vi "PH_BeamlineController.constructor.vi"(0 "name":string, 2 "data in":string, 5 "error in(no error)":errorcluster) -> (14 "i ref out":refnum<vi>, 16 "data out":string, 19 "error out":errorcluster)   [LabVIEW 2014, in "PH_BeamlineController.lvlib"]
doc: "The Sequencer controlles the PHELIX shot procedure.\n\nThis class is part of the PHELIX user layer.\n\nauthor: Stefan Götte, GSI\n\nLicense Agreement for this software:\n\nCopyright (C)\nGesellschaft für Schwerionenforschung, GSI\nPlanckstr. 1\n64291 Darmstadt\nGermany\n\nContact: D.Beck@gsi.de \n\nThis program is free software; you can redistribute it and/or modify it under the terms of the \nGNU General Public License as published by the Free Software Foundation; either version 2 of \nthe license, or (at your option) any later version.\n\nThis program is distributed in the hope that it will be useful, but WITHOUT ANY WARRANTY; \nwithout even the implied warranty of MERCHANTABILITY or FITNESS FOR A PARTICULAR PURPOSE. See the GNU General License for more details (http://www.gnu.org).\n\nGesellschaft für Schwerionenforschung, GSI\nPlanckstr. 1, 64291 Darmstadt, Germany\nFor all questions and ideas contact: M.Richter@gsi.de, H.Brand@gsi.de or D.Beck@gsi.de.\nLast update: 16-JUN-2004"
uses:
  PH_BeamlineController.lvlib
  PH_BeamlineInformation/PH_BeamlineInformation.lvlib
  CS_Core/CSSystem/CSSystemLib/CSSystemLib.lvlib
  PH_Basics/PH_Class/PH_Class.lvlib
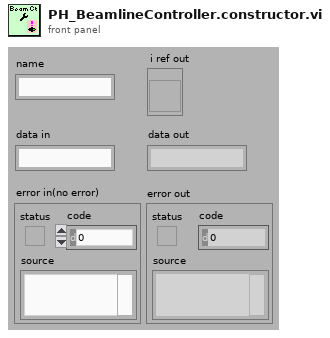
[diagram p1: front panel]
types:
  T1 = enum16{"SetAttribute", "GetAttribute", "CreateAttribute", "DestroyAttribute", "DestroyAllAtributes"}
  T2 = typedef "PH_BeamlineController.lvlib/PH_BeamlineController.i attribute.ctl" = cluster{"Vacuum Exp LB":cluster{"Channel":string, "Limit [mbar]":dbl, "Pressure [mbar]":dbl, "GUI Ref":refnum<vi>}, "Sources":T3[], "PA DP Targets":T5[], "Path":cluster{"Source":T4, "PA DP Target":T6, "Target":T7}, "Targets":cluster{"Name":T7, "GUI Ref":refnum<vi>, "Current State":bool, "Wanted State":bool, "Enabled":bool}[], "Status Tags":cluster{"Name":string, "Status":T8}[], "special GUI Refs":T9}
  T3 = typedef "PH_BeamlineController.lvlib/PH_BeamlineController.Source Attributes.ctl" = cluster{"Name":T4, "GUI Ref":refnum<vi>, "Current State":bool, "Wanted State":bool}
  T4 = typedef "PH_BeamlineController.lvlib/PH_BeamlineController.Sources.ctl" = enum16{"None", "YLF", "fs-Frontend", "ns-Frontend", "YLF and ns-Frontend", "fs- and ns-Frontend"}
  T5 = typedef "PH_BeamlineController.lvlib/PH_BeamlineController.PA DP Target Attributes.ctl" = cluster{"Name":T6, "GUI Ref":refnum<vi>, "Current State":bool, "Wanted State":bool, "Enabled":bool}
  T6 = typedef "PH_BeamlineController.lvlib/PH_BeamlineController.PA DP Targets.ctl" = enum16{"None", "Dump PA Delayed Beam", "Dump PA Undelayed Beam", "Dumps PA Delayed and Undelayed Beam"}
  T7 = typedef "PH_BeamlineController.lvlib/PH_BeamlineController.Targets.ctl" = enum16{"None", "PreAmp", "Dump Exp Laserlab", "Exp Laserlab", "Calorimeter", "Dump Exp Laserbay", "Exp Laserbay", "Dump Exp Z6", "Exp Z6"}
  T8 = typedef "PH_StatusHandler.lvlib/PH_StatusHandler.Status.ctl" = i16
  T9 = typedef "PH_BeamlineController.lvlib/PH_BeamlineController.special GUI Refs.ctl" = cluster{"PA-Backreflection-Meas":refnum<vi>, "fs_Synchrolock_Watch":refnum<vi>}
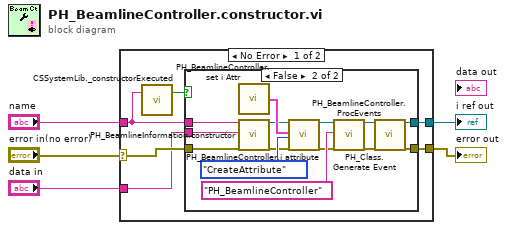
[diagram p0: block diagram]
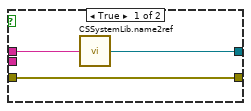
[diagram p2: hidden frame]
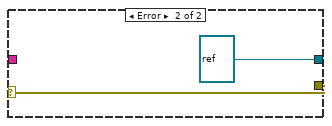
[diagram p3: hidden frame]
diagram:
  n1 = case shown="No Error" "error in(no error)" {
    selector: "error in(no error)" -> [w9 w30]
    tunnel: "name" -> [w8 _]
    tunnel: [w10 w30] -> w4
    tunnel: [w11 refnum<vi> refnum ("i ref out")] -> w3
    tunnel: "data in" -> [w6 _]
    frame No Error {
      n2 = call "CSSystemLib._constructorExecuted.vi"("name"=w8) -> ("constructor executed?"=w7:bool)  [unwired: 18 in]
      n3 = case shown="False" w7 {
        tunnel: [w12 w27] -> w11
        tunnel: [w14 w26] -> w10
        tunnel: w9 -> [w14 w15]
        tunnel: w8 -> [w13 w24]
        tunnel: w6 -> [_ w16]
        frame True {
          n4 = call "CSSystemLib.name2ref.vi"("name"=w13) -> ("obj refnum"=w12:refnum<vi>)
        }
        frame False {
          n5 = call "PH_BeamlineController.set i Attr.vi"() -> ("PH_BeamlineController.i attribute"=w25:T2)  [unwired: 1 in]
          n6 = call "PH_BeamlineInformation.constructor.vi"("name"=w24, "data in"=w16, "error in(no error)"=w15) -> ("i ref out"=w22:refnum<vi>, "error out"=w21:errorcluster)  [unwired: 14 in, 1 out]
          n7 = call "PH_BeamlineController.i attribute.vi"("VI Refnum"=w22, "CLASS.i attribute"=w25, "Action"=T1."CreateAttribute", "error in (no error)"=w21) -> ("VI Refnum out"=w20:refnum<vi>, "error out"=w18:errorcluster)  [unwired: 13 in, 1 out]
          n8 = call "PH_Class.Generate Event.vi"("i ref in"=w20, "Class"="PH_BeamlineController", "error in (no error)"=w18) -> ("i ref out"=w19:refnum<vi>, "error out"=w17:errorcluster)  [unwired: 15 in]
          n9 = call "PH_BeamlineController.ProcEvents.vi"("i ref in"=w19, "error in (no error)"=w17) -> ("i ref out"=w27:refnum<vi>, "error out"=w26:errorcluster)  [unwired: 16 in]
        }
      }
    }
    frame Error {
    }
  }
  "i ref out" <- w3
  "error out" <- w4
